vi "Write MeasurementDetails.vi"(8 "error in (no error)":errorcluster, 10 "ni_measurements_v1_MeasurementDetails":T1, 11 "MeasurementService in":refnum<class "MeasurementService.lvclass">) -> (0 "error out":errorcluster, 3 "MeasurementService out":refnum<class "MeasurementService.lvclass">)   [LabVIEW 2020, in "MeasurementTemplate_server.lvlib" / "MeasurementService.lvclass"]
uses:
  MeasurementService.lvclass
  RPC Messages/ni_measurements_v1_MeasurementDetails.ctl
  MeasurementService.lvclass/MeasurementService.ctl
  MeasurementTemplate_server.lvlib
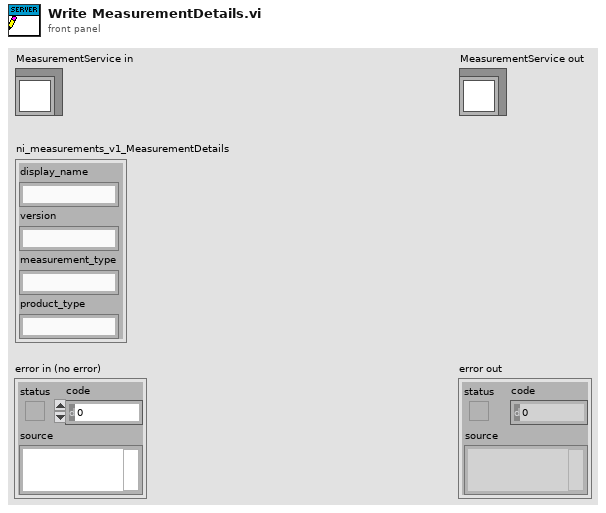
[diagram p1: front panel]
types:
  T1 = typedef "MeasurementTemplate_server.lvlib/ni_measurements_v1_MeasurementDetails.ctl" = cluster{"display_name":string, "version":string, "measurement_type":string, "product_type":string}
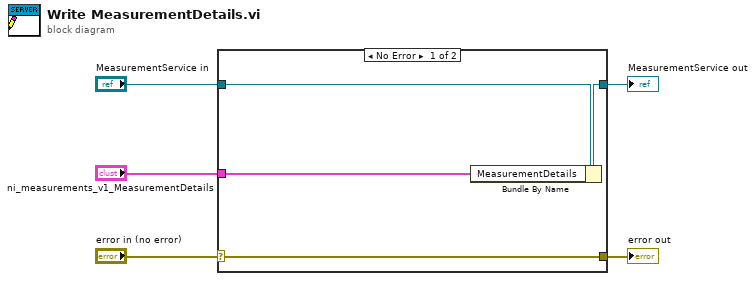
[diagram p0: block diagram]
diagram:
  n1 = case shown="No Error" "error in (no error)" {
    selector: "error in (no error)" -> [w9 w10]
    tunnel: [w9 w10] -> w4
    tunnel: [w7 w11] -> w2
    tunnel: "MeasurementService in" -> [w8 w11]
    tunnel: "ni_measurements_v1_MeasurementDetails" -> [w6 _]
    frame No Error {
      n2 = Bundle By Name(cluster=w8, "MeasurementDetails"=w6) -> (w7:refnum<class "MeasurementService.lvclass">)
    }
    frame Error {
    }
  }
  "error out" <- w4
  "MeasurementService out" <- w2
